vi "CMN_SeparateField.vi"(7 "field separator":string="[.]", 8 "error in (no error)":errorcluster, 10 "search parent":string, 11 "input arg":string) -> (0 "error out":errorcluster, 1 "found":bool, 2 "field":string, 3 "parent":string)   [LabVIEW 2016]
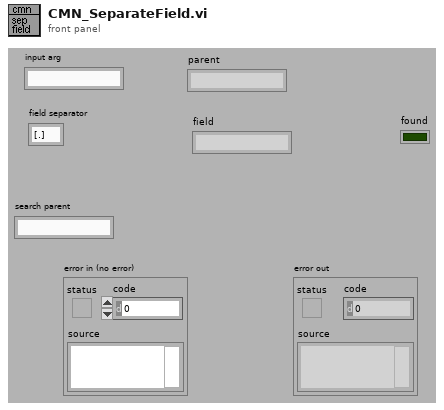
[diagram p1: front panel]
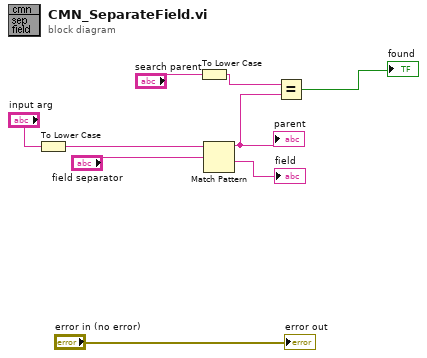
[diagram p0: block diagram]
diagram:
  n1 = To Lower Case(string="input arg") -> (all lower case string=w1:string)
  n2 = To Lower Case(string="search parent") -> (all lower case string=w2:string)
  n3 = Match Pattern(string=w1, regular expression="field separator") -> (before substring=w5:string, after substring=→"field":string)  [unwired: 3 out]
  "parent" <- w5
  n4 = Equal?(x=w2, y=w5) -> (x = y?=→"found":bool)
  "error out" <- "error in (no error)"
